vi "Advanced Single Point Benchmark.vi"() -> ()   [LabVIEW 2011]
panel:
  in  "Configuration:Measurement Options:DC Noise Rejection":i32(ring)=2 items=["Auto"=-1, "Normal"=0, "Second_Order"=1, "High_Order"=2]
  in  "Configuration:Advanced:Settle Time":dbl=0.001
  in  "Configuration:Advanced:Aperture Time":dbl=0.1
  in  "Configuration:Advanced:Aperture Time Units":i32(ring) items=["NIDMM_VAL_SECONDS", "NIDMM_VAL_POWER_LINE_CYCLES"]
  in  "Configuration:Function":i32(ring)=1 items=["NIDMM_VAL_DC_VOLTS"=1, "NIDMM_VAL_AC_VOLTS"=2, "NIDMM_VAL_DC_CURRENT"=3, "NIDMM_VAL_AC_CURRENT"=4, "NIDMM_VAL_2_WIRE_RES"=5, "NIDMM_VAL_4_WIRE_RES"=101, "NIDMM_VAL_FREQ"=104, "NIDMM_VAL_PERIOD"=105, "NIDMM_VAL_AC_VOLTS_DC_COUPLED"=1001, "NIDMM_VAL_DIODE"=1002, "NIDMM_VAL_CAPACITANCE"=1005, "NIDMM_VAL_INDUCTANCE"=1006, "NIDMM_VAL_WAVEFORM_VOLTAGE"=1003, "NIDMM_VAL_WAVEFORM_CURRENT"=1004]
  in  "Configuration:Range":dbl=10.0
  in  "Configuration:Measurement Options:ADC Calibration":i32(ring)=1 items=["Auto"=-1, "Off"=0, "On"=1]
  in  "Configuration:Measurement Options:Auto Zero":i32(ring)=1 items=["Auto"=-1, "Off"=0, "On"=1, "Once"=2]
  out "Measurement Period (seconds)":dbl format="%.4f"
  in  "Instrument Descriptor":refnum<k15>="DMM"
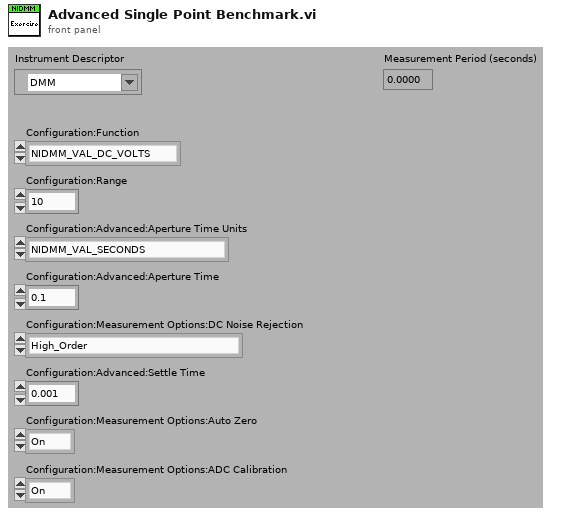
[diagram p1: front panel]
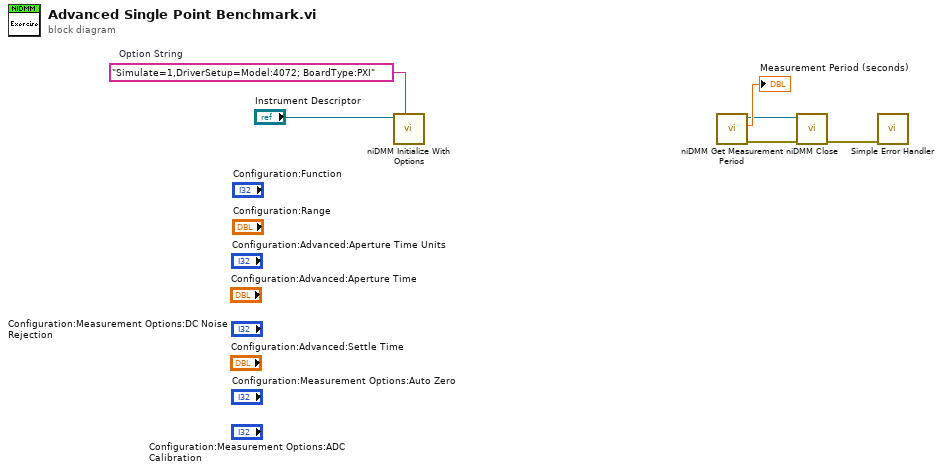
[diagram p0: block diagram]
diagram:
  w1 = "Simulate=1,DriverSetup=Model:4072; BoardType:PXI"  # Option String
  n1 = call <instrlib>:"niDMM Initialize With Options.vi"("Option String"=w1, "Instrument Descriptor"="Instrument Descriptor") -> ()  [unwired: 8 in, 2 out]
  n2 = call <instrlib>:"niDMM Get Measurement Period.vi"() -> ("error out"=w4:errorcluster, "Measurement Period (seconds)"=→"Measurement Period (seconds)":dbl, "instrument handle out"=w3:refnum<k15>)  [unwired: 9 in]
  n3 = call <instrlib>:"niDMM Close.vi"("error in (no error)"=w4, "instrument handle"=w3) -> ("error out"=w2:errorcluster)  [unwired: 9 in]
  n4 = call <vilib>:"Simple Error Handler.vi"("error in (no error)"=w2) -> ()  [unwired: 4 in, 5 out]
